vi "Init.vi"(8 "error in (no error)":errorcluster) -> (0 "error out":errorcluster, 3 "Logging out":refnum<class "Logging.lvclass">)   [LabVIEW 2020, in "Logging.lvclass"]
uses:
  Logging.lvclass
  controls/Log entry.ctl
  Logging.lvclass/Logging.ctl
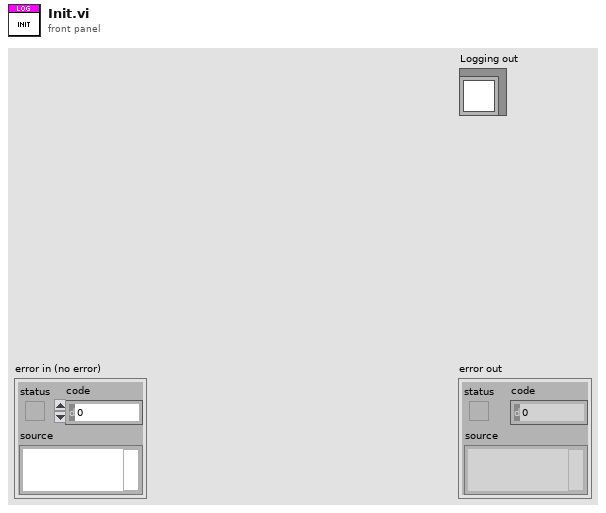
[diagram p1: front panel]
types:
  T1 = typedef "Log entry.ctl" = cluster{"timestamp":timestamp, "data":variant, "origin":string, "severity":i32}
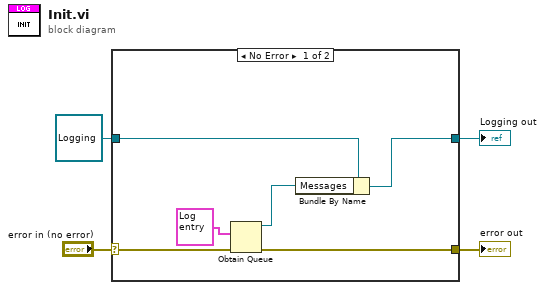
[diagram p0: block diagram]
diagram:
  n1 = case shown="No Error" "error in (no error)" {
    selector: "error in (no error)" -> [w7 w12]
    tunnel: [w6 w12] -> w3
    tunnel: [w10 w11] -> w1
    tunnel: refnum<class "Logging.lvclass"> refnum ("Logging in") -> [w5 w11]
    frame No Error {
      n2 = Obtain Queue(element data type=T1 {"timestamp"=timestamp(0 s since 1904-01-01), "data"=variant, "origin"="", "severity"=0} ("Log entry"), error in (no error)=w7) -> (queue out=w9:refnum<queue>, error out=w6:errorcluster)  [unwired: 3 in, 1 out]
      n3 = Bundle By Name(cluster=w5, "Messages"=w9) -> (w10:refnum<class "Logging.lvclass">)
    }
    frame Error {
    }
  }
  "error out" <- w3
  "Logging out" <- w1
